vi "Send List of Measurements Message.vi"(8 "error in (no error)":errorcluster, 10 "List of Measurement Names":string[](array[string]), 11 "Message Enqueuer in":refnum<class "Message Enqueuer.lvclass">) -> (0 "error out":errorcluster, 3 "Message Enqueuer out":refnum<class "Message Enqueuer.lvclass">)   [LabVIEW 2015, in "Measurement UI.lvlib" / "List of Measurements Message.lvclass"]
uses:
  List of Measurements Message.lvclass
  <vilib>/ActorFramework/Message Enqueuer/Message Enqueuer.lvclass
  <vilib>/ActorFramework/Message Enqueuer/Message Enqueuer.lvclass/Message Enqueuer.ctl
  <vilib>/ActorFramework/Message Priority Queue/Priority Enqueue.vi
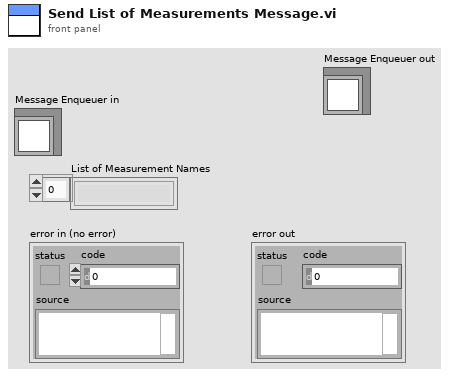
[diagram p1: front panel]
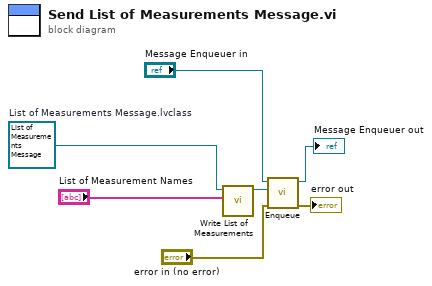
[diagram p0: block diagram]
diagram:
  w7 = refnum<class "List of Measurements Message.lvclass"> refnum  # List of Measurements Message.lvclass
  n1 = call "Write List of Measurements.vi"("List of Measurements"="List of Measurement Names", "List of Measurements Message in"=w7) -> ("List of Measurements Message out"=w3:refnum<class "List of Measurements Message.lvclass">)  [unwired: 8 in, 1 out]
  n2 = call <vilib>:"Enqueue.vi"("error in (no error)"="error in (no error)", "Message"=w3, "Message Enqueuer in"="Message Enqueuer in") -> ("error out"=→"error out":errorcluster, "Message Enqueuer out"=→"Message Enqueuer out":refnum<class "Message Enqueuer.lvclass">)  [unwired: 7 in]
